vi "点距离.vi"(0 "二维点阵":cluster{"X":sgl, "Y":sgl}[][](array[cluster])) -> (1 "X间距":sgl, 2 "Y间距":sgl)   [LabVIEW 2018]
uses:
  <vilib>/vision/NI_Vision_Development_Module.lvlib
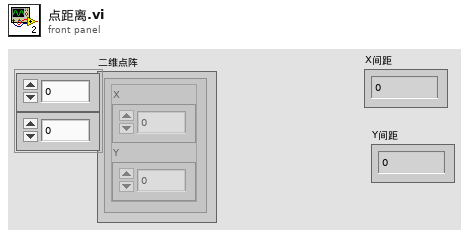
[diagram p1: front panel]
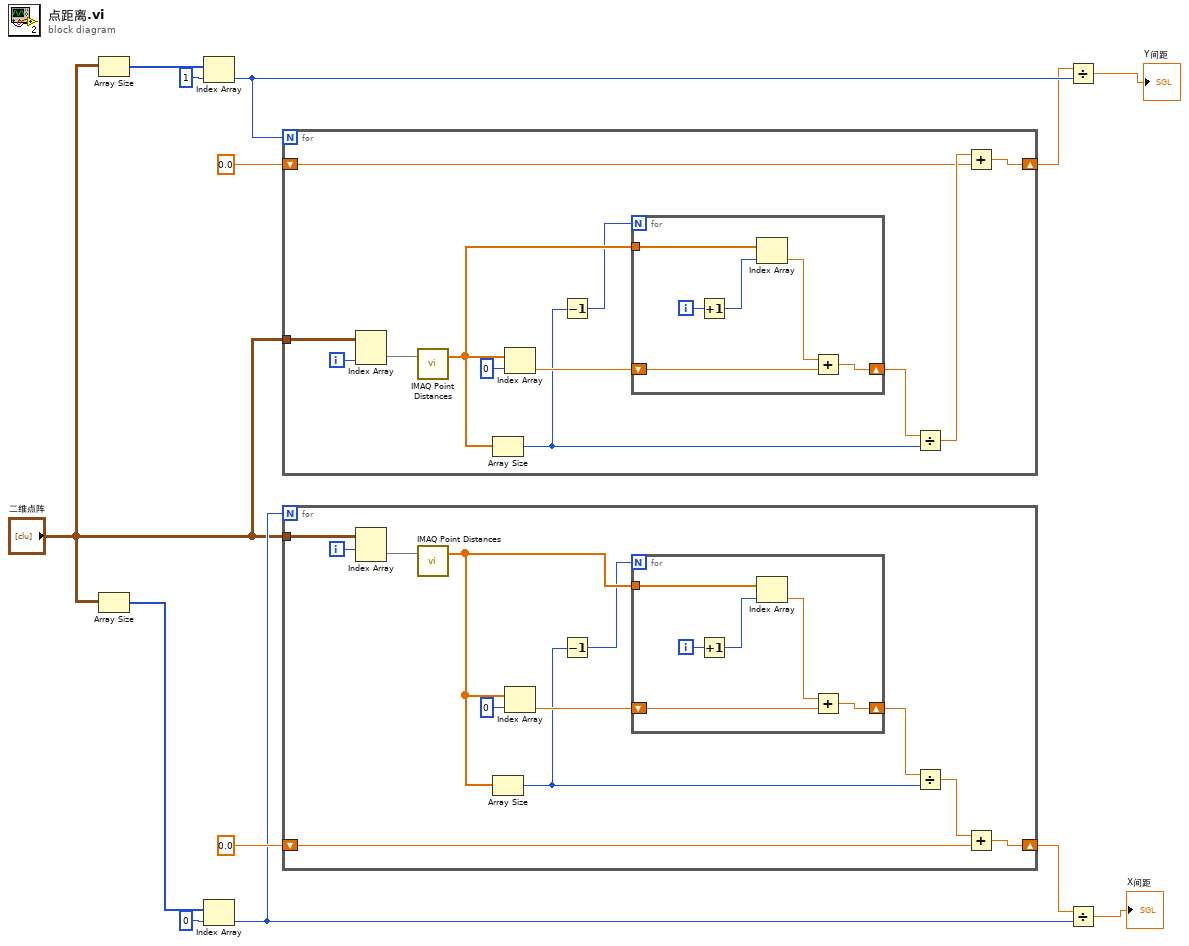
[diagram p0: block diagram]
diagram:
  n1 = Array Size(array="二维点阵") -> (size(s)=w4:i32[])
  n2 = Array Size(array="二维点阵") -> (size(s)=w13:i32[])
  n3 = Index Array(array=w4, index=1 ("索引")) -> (element=w8:i32)
  n4 = Index Array(array=w13, index=0 ("索引")) -> (element=w9:i32)
  n5 = for {
    N: w8 -> [_]
    tunnel: "二维点阵" -> [w25]
    shift-right: [w17] -> w7
    shift-left: sgl 0.0 -> [w16]
    i -> [w14]
    n6 = Index Array(array=w25, index (col)=w14) -> (element=w24:cluster{"X":sgl, "Y":sgl}[])  [unwired: 1 in]
    n7 = call "IMAQ Point Distances"("Points"=w24) -> ("Distances"=w22:sgl[])  [unwired: 4 in, 1 out]
    n8 = Array Size(array=w22) -> (size(s)=w15:i32)
    n9 = Index Array(array=w22, index=0 ("索引")) -> (element=w21:sgl)
    n10 = Decrement(x=w15) -> (x-1=w19:i32)
    n11 = for {
      N: w19 -> [_]
      tunnel: w22 -> [w31]
      shift-right: [w26] -> w20
      shift-left: w21 -> [w27]
      i -> [w30]
      n12 = Increment(x=w30) -> (x+1=w29:i32)
      n13 = Index Array(array=w31, index=w29) -> (element=w28:sgl)
      n14 = Add(x=w28, y=w27) -> (x+y=w26:sgl)
    }
    n15 = Divide(x=w20, y=w15) -> (x/y=w18:sgl)
    n16 = Add(x=w18, y=w16) -> (x+y=w17:sgl)
  }
  n17 = for {
    N: w9 -> [_]
    tunnel: "二维点阵" -> [w43]
    shift-right: [w34] -> w10
    shift-left: sgl 0.0 -> [w33]
    i -> [w42]
    n18 = Index Array(array=w43, index (row)=w42) -> (element=w41:cluster{"X":sgl, "Y":sgl}[])  [unwired: 1 in]
    n19 = call "IMAQ Point Distances"("Points"=w41) -> ("Distances"=w39:sgl[])  [unwired: 4 in, 1 out]
    n20 = Array Size(array=w39) -> (size(s)=w32:i32)
    n21 = Index Array(array=w39, index=0 ("索引")) -> (element=w38:sgl)
    n22 = Decrement(x=w32) -> (x-1=w36:i32)
    n23 = for {
      N: w36 -> [_]
      tunnel: w39 -> [w49]
      shift-right: [w44] -> w37
      shift-left: w38 -> [w45]
      i -> [w48]
      n24 = Increment(x=w48) -> (x+1=w47:i32)
      n25 = Index Array(array=w49, index=w47) -> (element=w46:sgl)
      n26 = Add(x=w46, y=w45) -> (x+y=w44:sgl)
    }
    n27 = Divide(x=w37, y=w32) -> (x/y=w35:sgl)
    n28 = Add(x=w35, y=w33) -> (x+y=w34:sgl)
  }
  n29 = Divide(x=w7, y=w8) -> (x/y=→"Y间距":sgl)
  n30 = Divide(x=w10, y=w9) -> (x/y=→"X间距":sgl)
